vi "SDCP - Read Parameter From Frame.vi"(2 "error in (no error)":errorcluster, 3 "Parameter":string) -> (0 "error out":errorcluster, 1 "Value":dbl)   [LabVIEW 2020]
uses:
  Typedefs/SDCP - Standard Message Frame Parameters - FGV - commands.ctl
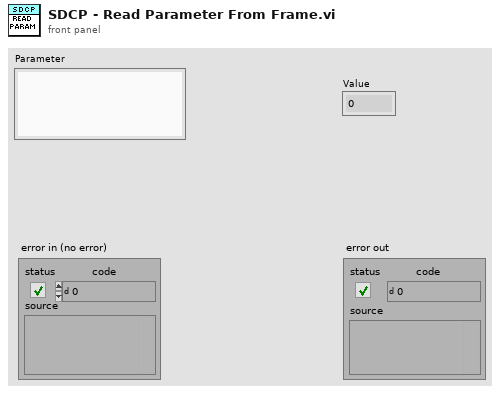
[diagram p1: front panel]
types:
  T1 = typedef "SDCP - Standard Message Frame Parameters - FGV - commands.ctl" = enum16{"Write descriptors", "Read descriptors", "Read values", "Load parameters from file", "Write values", "Read all descriptors"}
  T2 = typedef "SDCP - SMF parameter descriptors.ctl" = cluster{"Frame name":string, "Frame ID":i32, "Data type":string, "Start Position":i32, "Length":i32, "Factor":dbl, "Offset":dbl, "Parameter name":string, "Value":string}
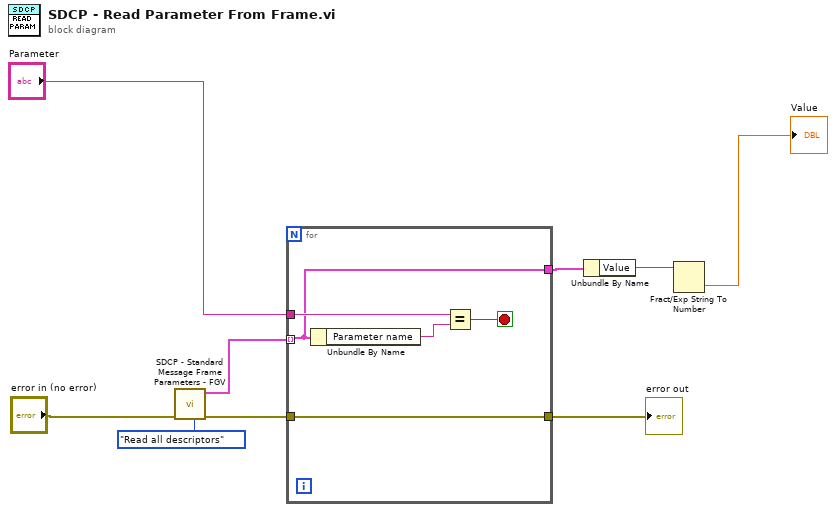
[diagram p0: block diagram]
diagram:
  n1 = call "SDCP - Standard Message Frame Parameters - FGV.vi"("error in (no error)"="error in (no error)", "Command"=SDCP_-_Standard_Message_Frame_Parameters_-_FGV_-_commands."Read all descriptors") -> ("SMF Parameters descriptors out"=w6:T2[], "error out"=w7:errorcluster)  [unwired: 5 in]
  n2 = for {
    tunnel: w7 -> [w11]
    tunnel: w6 -> [w10] mode=indexing
    tunnel: "Parameter" -> [w13]
    tunnel: [w11] -> w1
    tunnel: [w10] -> w4
    stop <- w12 stop-if-true
    n3 = Unbundle By Name(w10) -> ("Parameter name"=w14:string)
    n4 = Equal?(x=w13, y=w14) -> (x = y?=w12:bool)
  }
  "error out" <- w1
  n5 = Unbundle By Name(w4) -> ("Value"=w3:string)
  n6 = Fract/Exp String To Number(string=w3) -> (number=→"Value":dbl)  [unwired: 3 in, 1 out]
